vi "Patterns analysis.vi"() -> ()   [LabVIEW 2020, in "AoC 2022.lvlib"]
uses:
  AoC 2022.lvlib
panel:
  out "Array":T1(array[cluster])
  in  "map":T2(c390)
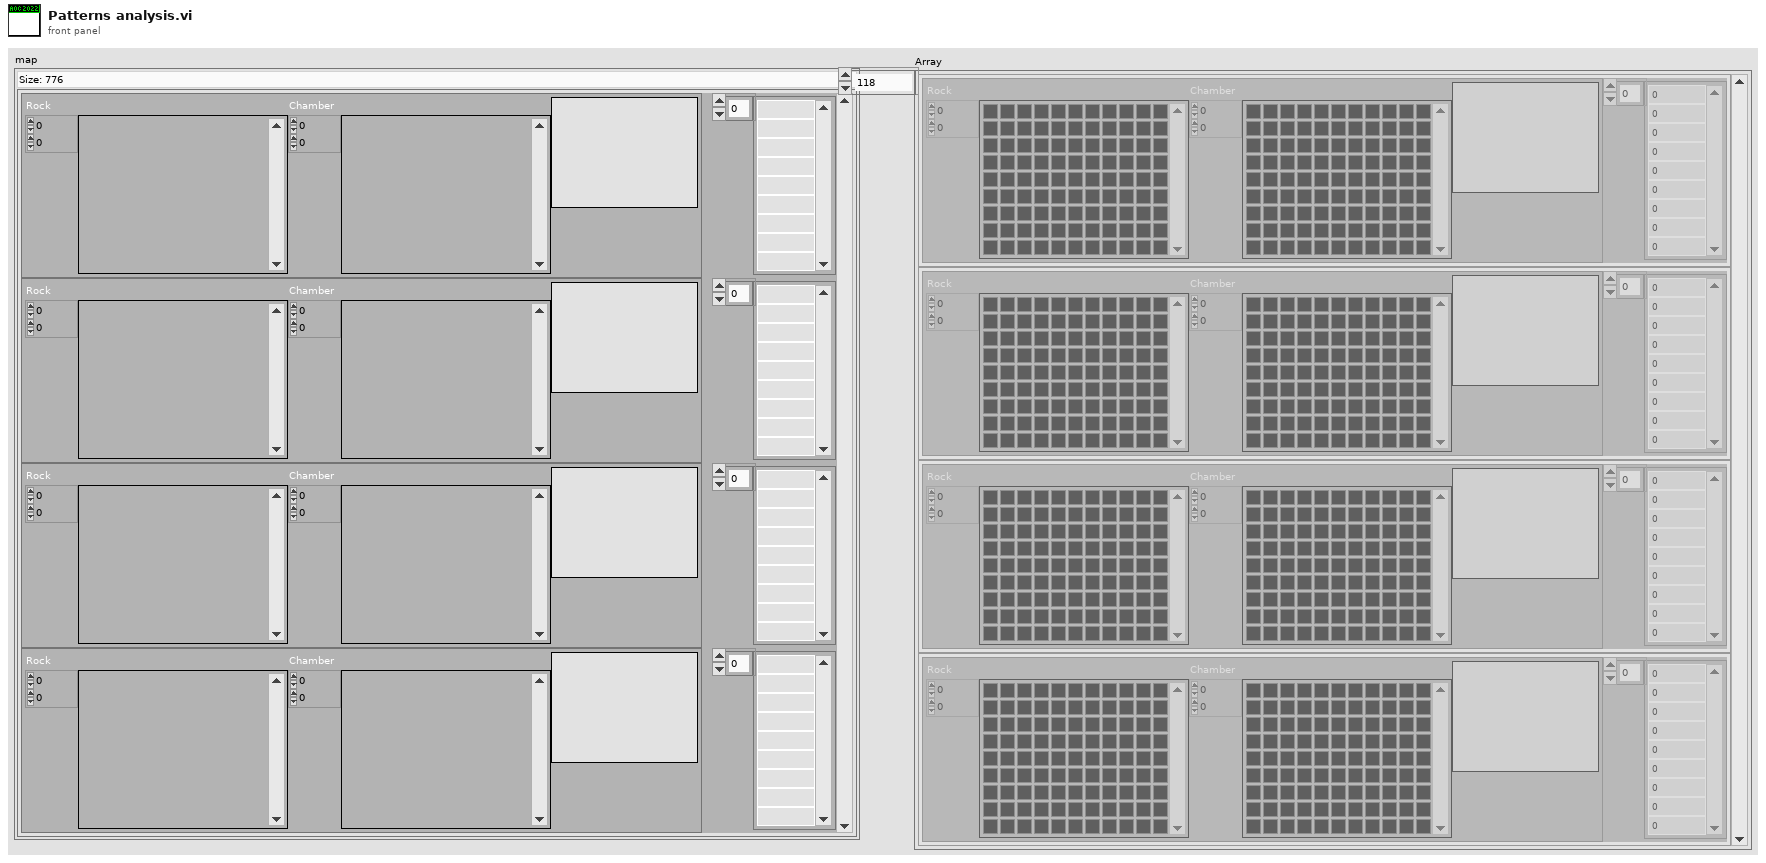
[diagram p1: front panel]
types:
  T1 = cluster{"key":cluster{"Rock":u32[][], "Chamber":u32[][], string}, "value":i32[]}[]
  T2 = map{cluster{"Rock":u32[][], "Chamber":u32[][], string}, i32[]}
  T3 = cluster{"Rock":u32[][], "Chamber":u32[][], string}
  T4 = cluster{"key":cluster{"Rock":u32[][], "Chamber":u32[][], string}, i32[]}
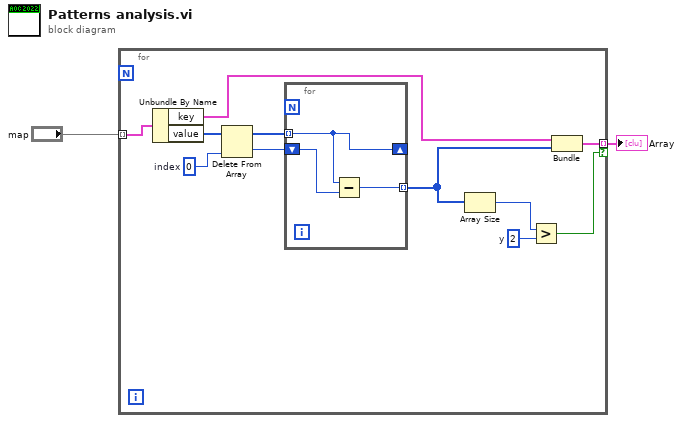
[diagram p0: block diagram]
diagram:
  n1 = for {
    tunnel: "map" -> [w13] mode=indexing
    tunnel: [w7] -> w1 mode=indexing if=w3
    w4 = 2  # y
    w9 = 0  # index
    n2 = Unbundle By Name(w13) -> ("key"=w8:T3, "value"=w12:i32[])
    n3 = Delete From Array(array=w12, index=w9) -> (deleted portion=w10:i32, array with subset deleted=w11:i32[])  [unwired: 1 in]
    n4 = for {
      tunnel: w11 -> [w15] mode=indexing
      shift-right: [w15] -> _
      shift-left: w10 -> [w16]
      tunnel: [w14] -> w6 mode=indexing
      n5 = Subtract(x=w15, y=w16) -> (x-y=w14:i32)
    }
    n6 = Array Size(array=w6) -> (size(s)=w5:i32)
    n7 = Greater?(x=w5, y=w4) -> (0:w3:bool)
    n8 = Bundle("key"=w8, w6) -> (w7:T4)  [unwired: 1 in]
  }
  "Array" <- w1
